vi "Select Component.vi"(7 "Disable Others?":T1, 8 "error in (no error)":errorcluster, 10 "Component":string, 11 "Camera in":refnum<class "Camera.lvclass">) -> (0 "error out":errorcluster, 3 "Camera":refnum<class "Camera.lvclass">)   [LabVIEW 2020, in "Camera.lvclass"]
uses:
  Camera.lvclass
  Component Selection Mode.ctl
  Camera.lvclass/Camera.ctl
  bin/gindustrialcam_32-1.dll
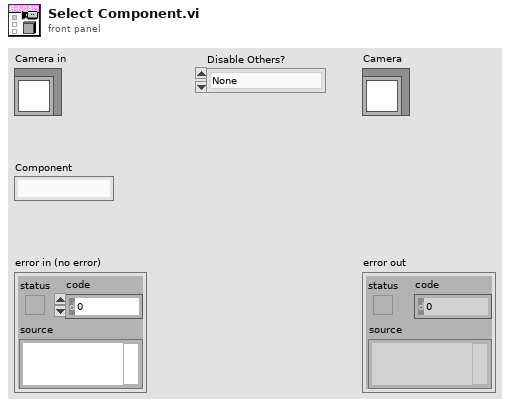
[diagram p1: front panel]
types:
  T1 = typedef "Camera.lvclass/Component Selection Mode.ctl" = enum8{"None", "Enable", "Disable", "Exclusive Enable", "Enable All"}
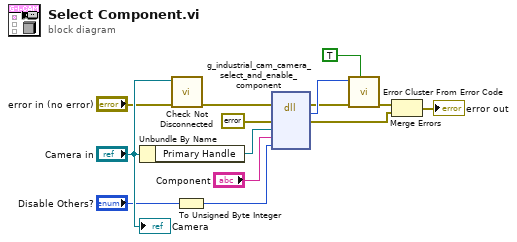
[diagram p0: block diagram]
diagram:
  n1 = Unbundle By Name("Camera in") -> ("Primary Handle"=w9:refnum<data-value>)
  n2 = call "Check Not Disconnected.vi"("error in (no error)"="error in (no error)", "Camera in"="Camera in") -> ("error out"=w10:errorcluster)  [unwired: 9 in]
  n3 = To Unsigned Byte Integer(number="Disable Others?") -> (unsigned 8bit integer=w1:u8)
  n4 = dll-call lib="C:/serenial/lib/g-industrial-camera/LabVIEW/g_industrial_cam/bin/gindustrialcam_*-1.*" fn="g_industrial_cam_camera_select_and_enable_component"(error in=w10, "err"=errorcluster {"status"=FALSE, "code"=0, "source"=""} ("error constant"), "edvr"=w9, "component"="Component", "selection_mode"=w1) -> (error out=w3:errorcluster, "Mg_Error"=w4:i32, "err"=w6:errorcluster)  [unwired: 5 in, 1 out]
  n5 = call <vilib>:"Error Cluster From Error Code.vi"("show call chain? (False)"=TRUE, "error in (no error)"=w3, "error code (0)"=w4) -> ("error out"=w5:errorcluster)  [unwired: 6 in]
  n6 = Merge Errors(w5, w6) -> (→"error out":errorcluster)
  "Camera" <- "Camera in"
